vi "UDP Sender.vi"(4 "error in":errorcluster, 5 "Show panel":bool, 6 "boost":dbl=1.0, 7 "Spot Params":T1=[{"Intensity"=1.0, "Vortex"=0.0, "Phase"=0.0, "X"=4.0, "Y"=0.0, "Z"=0.0}, {"Intensity"=0.0, "Vortex"=0.0, "Phase"=0.0, "X"=-7.0, "Y"=6.0, "Z"=0.0}] {"Z" format="%_4g"; "Y" format="%_4g"; "X" format="%_4g"; "Phase" format="%_4g"; "Intensity" format="%_4g"}) -> (0 "error out":errorcluster, 3 "length":i32=234)   [LabVIEW 2020]
doc: "This VI sends UDP packets to the hologram server so that it can display holograms. It also has a lot of settings on the front panel, which control most of the aspects of hologram generation and display."
uses:
  <vilib>/Analysis/Matrix/Datatypes/RealMatrix.ctl
  _Controls/Spot Params.ctl
  <vilib>/Analysis/Matrix/NI_Matrix.lvlib
panel:
  in  "NA Position":cluster{"x":dbl, "y":dbl, "r":dbl}={"x"=0.0, "y"=0.0, "r"=1.0}
  in  "Save settings to defaults file":bool
  in  "SLM Settings":T2(tab)=enum."Scaling Factors"
  in  "Remote Host":string="127.0.0.1"
  in  "Local Port":u16=61556
  in  "Remote Port":u16=61557
  in  "-¹..¹ range control":enum16{"wrap round", "cast to range"}(ring)=enum."cast to range"
  out "'blazing function'":cluster{dbl, dbl}[](graph)=[{-3.141592653589793, 0.0}, {-2.938909256584, 0.057923902564858604}, {-2.736225859578207, 0.11496236941997928}, {-2.533542462572414, 0.1702299648556241}, {-2.330859065566621, 0.22284125316205516}, {-2.1281756685608277, 0.2719107986295345}, {-1.9254922715550344, 0.31655316554832424}, {-1.7228088745492414, 0.3558829182086864}, {-1.5201254775434483, 0.38901462090088307}, {-1.317442080537655, 0.41506283791517634}, {-1.114758683531862, 0.4334376236022463}, {-0.9120752865260688, 0.44502212608587055}, {-0.7093918895202758, 0.4511576344794046}, {-0.5067084925144827, 0.4531855832933398}, {-0.3040250955086896, 0.45244740703816744}, {-0.10134169850289654, 0.4502845402243789}, {0.10134169850289654, 0.44803841736246536}, {0.30402509550868917, 0.44705047296291806}, {0.5067084925144831, 0.44866214153622835}, {0.7093918895202758, 0.45421485759288766}, {0.9120752865260693, 0.46505005564338703}, {1.1147586835318615, 0.48250917019821804}, {1.3174420805376554, 0.5079336357678718}, {1.5201254775434485, 0.5426266162553631}, {1.7228088745492416, 0.5867222378526288}, {1.9254922715550338, 0.6389982972954518}, {2.1281756685608277, 0.6981566028735295}, {2.330859065566621, 0.7628989628765593}, {2.533542462572414, 0.8319271855942384}, {2.736225859578207, 0.9039430793162642}, {2.938909256584, 0.9776484523323339}, {3.141592653589793, 1.0}]
  in  "Hologram location on-screen":T3={"Display Mode"=0, "Coordinates (x,y,width,height)"=[2560, 0, 512, 512]} {"Display Mode" items=["Coordinates given below", "All of monitor 1", "All of monitor 2", "All of monitor 3", "All of monitor 4", "All of monitor 5"]}
  in  "Aspect Ratio and Centering":T4={"Physical Aspect Ratio (width/height)"=1.0, "Screen Aspect Ratio (width in pixels/height in pixels)"=1.0, "Illumination Centre (range: 0 to 1)"={"x"=0.49, "y"=0.52}} {"Illumination Centre (range: 0 to 1)"."y" min=0.0 max=1.0 step=0.001; "Illumination Centre (range: 0 to 1)"."x" min=0.0 max=1.0 step=0.001}
  in  "Zernike Coefficients":dbl[](array[numeric])=[1.0, 0.0, -1.0, 0.0, 0.0, 0.0, 0.0, 0.0, 0.0, 0.0, 0.0, 0.0]
  in  "Enable":bool=TRUE
  in  "Multiplier":dbl=10.0
  out "Phase Map":dbl[][](graph)=[[1.1504440784612413, 1.1088207694081724, 0.9839508422489622, 0.7758342969836143, 0.484471133612125, 0.10986135213450154, -0.3479950474492668, -0.8890980651391764, -1.5134477009352203, -2.2210439548374055, -3.0118868268457284, 2.39720899021939, 1.439872881998788, 0.39929015567204473, -0.7245391887608363, -1.9316151512998605, 3.0612475752345656, 1.6876783764832677, 0.23086255962582847, -1.3091998753377538, -2.932508928407473, 1.6441207075962554, -0.1456815816857464, -2.0187304890738824, 2.308159292611429, 0.2686171490110141, -1.8541716126955379, 2.222978314671346, -0.06630368324748659, -2.438832299272459, 1.38857777377601, -1.1504440784612413], [-1.38857777377601, -1.3469544647229412, -1.38857777377601, -1.5134477009352203, -1.7215642462005682, -2.0129274095720575, -2.387537191049681, -2.8453935906334493, 2.8966886988562273, 2.2723390630601834, 1.5647428091579982, 0.7738999371496718, -0.1001895529647907, -1.0575256611853927, -2.098108387512136, 3.0612475752345656, 1.8541716126955432, 0.5638490320503848, -0.8097201667009148, -2.2665359835583576, 2.476586888657649, 0.8532778355879307, -0.8532778355879307, -2.643080124869927, 1.767056274921524, -0.1892392505727507, -2.2287813941731667, 1.9316151512998587, -0.27442022851283454, -2.563702226431669, 1.3469544647229412, -1.1088207694081724], [2.438832299272459, 2.563702226431669, 2.6053255354847416, 2.563702226431669, 2.438832299272459, 2.230715754007111, 1.9393525906356253, 1.5647428091579947, 1.10688640957423, 0.5657833918843238, -0.05856624391172183, -0.766162497813907, -1.5570053698222317, -2.431094859936694, 2.8947543390222865, 1.8541716126955432, 0.7303422682626604, -0.4767336942763585, -1.7670562749215186, -3.1406254736728236, 1.6857440166493252, 0.1456815816857464, -1.477627471383978, 3.099002164619751, 1.3091998753377556, -0.5638490320503795, -2.520144557544656, 1.723498606034509, -0.39929015567204296, -2.605325535484738, 1.38857777377601, -0.9839508422489622], [0.06630368324748659, 0.27442022851283454, 0.39929015567204473, 0.44091346472511006, 0.3992901556720412, 0.27442022851283454, 0.06630368324748659, -0.22505948012400268, -0.5996692616016315, -1.0575256611853963, -1.5986286788753024, -2.222978314671348, -2.930574568573535, 2.5617678665977284, 1.6876783764832641, 0.7303422682626604, -0.31024045806408296, -1.434069802496964, -2.6411457650359838, 2.351716961498438, 0.9781477627471382, -0.478668054110301, -2.0187304890738833, 2.6411457650359846, 0.9345900938601268, -0.8552121954218688, -2.7282611028100057, 1.5986286788753006, -0.44091346472511184, -2.5637022264316656, 1.5134477009352203, -0.7758342969836143], [-2.222978314671346, -1.9316151512998587, -1.723498606034509, -1.5986286788753006, -1.5570053698222317, -1.5986286788753006, -1.7234986060345108, -1.9316151512998587, -2.222978314671346, -2.597588096148975, -3.05544449573274, 2.6866377937569386, 2.062288157960893, 1.3546919040587078, 0.5638490320503848, -0.31024045806408296, -1.267576566284685, -2.3081592926114256, 2.8511966701352787, 1.6441207075962545, 0.35379812695109436, -1.0197710718002062, -2.476586888657649, 2.2665359835583576, 0.6432269304886411, -1.063328740687215, -2.8531310299692105, 1.5570053698222317, -0.3992901556720412, -2.438832299272459, 1.7215642462005682, -0.484471133612125], [1.8541716126955468, 2.228781394173174, 2.5201445575446613, 2.728261102810009, 2.8531310299692194, 2.8947543390222883, 2.8531310299692194, 2.728261102810009, 2.5201445575446613, 2.228781394173174, 1.854171612695545, 1.3963152131117766, 0.8552121954218705, 0.2308625596258267, -0.4767336942763585, -1.267576566284685, -2.1416660563991483, -3.099002164619751, 2.1436004162330935, 1.019771071800208, -0.18730489073881262, -1.4776274713839723, -2.8511966701352773, 1.9751728201868701, 0.4351103852232914, -1.188198667846426, -2.894754339022281, 1.5986286788753006, -0.27442022851283454, -2.230715754007111, 2.0129274095720575, -0.10986135213450154], [-0.2686171490110123, 0.18923925057275603, 0.5638490320503831, 0.8552121954218705, 1.0633287406872185, 1.1881986678464287, 1.2298219768994976, 1.1881986678464287, 1.0633287406872185, 0.8552121954218705, 0.5638490320503813, 0.18923925057275426, -0.2686171490110123, -0.8097201667009166, -1.434069802496964, -2.141666056399149, -2.932508928407474, 2.47658688865765, 1.519250780437047, 0.47866805411030144, -0.6451612903225801, -1.8522372528616007, 3.14062547367282, 1.7670562749215213, 0.31024045806408207, -1.2298219768994958, -2.8531310299692123, 1.7234986060345108, -0.06630368324748659, -1.9393525906356235, 2.387537191049681, 0.3479950474492668], [-2.308159292611429, -1.767056274921524, -1.3091998753377556, -0.9345900938601268, -0.6432269304886411, -0.4351103852232914, -0.31024045806408296, -0.2686171490110123, -0.31024045806408296, -0.4351103852232914, -0.6432269304886411, -0.9345900938601286, -1.3091998753377556, -1.7670562749215213, -2.3081592926114283, -2.932508928407474, 2.643080124869927, 1.8522372528616033, 0.97814776274714, 0.020811654526533996, -1.0197710718002075, -2.143600416233089, 2.932508928407472, 1.642186347762312, 0.2686171490110123, -1.188198667846426, -2.728261102810004, 1.9316151512998587, 0.22505948012400268, -1.564742809157993, 2.8453935906334493, 0.8890980651391764], [2.0187304890738824, 2.643080124869927, -3.099002164619751, -2.6411457650359846, -2.2665359835583576, -1.9751728201868701, -1.7670562749215213, -1.642186347762312, -1.6005630387092422, -1.642186347762312, -1.7670562749215222, -1.9751728201868701, -2.2665359835583576, -2.6411457650359855, -3.099002164619752, 2.643080124869927, 2.0187304890738815, 1.3111342351716972, 0.5202913631633734, -0.3537981269510926, -1.311134235171696, -2.3517169614984375, 2.8076390012482637, 1.6005630387092422, 0.31024045806408296, -1.0633287406872167, -2.520144557544656, 2.222978314671346, 0.5996692616016315, -1.1068864095742263, -2.896688698856229, 1.5134477009352203], [0.1456815816857464, 0.8532778355879307, 1.477627471383978, 2.0187304890738833, 2.476586888657649, 2.851196670135277, -3.14062547367282, -2.932508928407472, -2.8076390012482637, -2.766015692195194, -2.8076390012482637, -2.932508928407473, -3.140625473672822, 2.851196670135277, 2.476586888657649, 2.0187304890738815, 1.4776274713839754, 0.8532778355879307, 0.14568158168574596, -0.645161290322581, -1.5192507804370443, -2.4765868886576468, 2.766015692195194, 1.642186347762312, 0.4351103852232914, -0.8552121954218688, -2.2287813941731685, 2.597588096148975, 1.0575256611853963, -0.565783391884322, -2.2723390630601834, 2.2210439548374055], [-1.6441207075962527, -0.8532778355879289, -0.14568158168574463, 0.4786680541103028, 1.019771071800208, 1.4776274713839754, 1.8522372528616033, 2.143600416233091, 2.3517169614984397, 2.476586888657648, 2.5182101977107187, 2.476586888657648, 2.3517169614984397, 2.1436004162330917, 1.8522372528616025, 1.4776274713839754, 1.0197710718002089, 0.4786680541103028, -0.14568158168574197, -0.8532778355879294, -1.6441207075962532, -2.5182101977107165, 2.8076390012482637, 1.7670562749215222, 0.6432269304886402, -0.5638490320503804, -1.8541716126955414, 3.05544449573274, 1.5986286788753024, 0.05856624391172538, -1.5647428091579982, 3.01188682684573], [2.932508928407473, -2.476586888657649, -1.6857440166493252, -0.9781477627471382, -0.35379812695109436, 0.18730489073881262, 0.6451612903225801, 1.019771071800207, 1.3111342351716964, 1.5192507804370443, 1.6441207075962527, 1.6857440166493234, 1.6441207075962536, 1.5192507804370443, 1.3111342351716964, 1.019771071800208, 0.6451612903225805, 0.1873048907388144, -0.35379812695109125, -0.9781477627471387, -1.6857440166493232, -2.476586888657647, 2.932508928407473, 1.9751728201868701, 0.9345900938601286, -0.18923925057275248, -1.396315213111774, -2.6866377937569386, 2.222978314671348, 0.7661624978139105, -0.7738999371496718, -2.39720899021939], [1.3091998753377547, 2.2665359835583576, 3.1406254736728236, -2.3517169614984375, -1.644120707596254, -1.019771071800208, -0.47866805411030144, -0.020811654526533996, 0.3537981269510926, 0.645161290322581, 0.8532778355879294, 0.9781477627471382, 1.019771071800208, 0.9781477627471382, 0.8532778355879294, 0.645161290322581, 0.35379812695109303, -0.02081165452653444, -0.478668054110301, -1.019771071800208, -1.6441207075962536, -2.351716961498438, 3.140625473672822, 2.2665359835583576, 1.3091998753377556, 0.2686171490110141, -0.8552121954218679, -2.062288157960893, 2.930574568573535, 1.5570053698222335, 0.1001895529647907, -1.439872881998788], [-0.23086255962582225, 0.8097201667009184, 1.767056274921524, 2.641145765035988, -2.8511966701352747, -2.14360041623309, -1.5192507804370434, -0.9781477627471373, -0.5202913631633708, -0.14568158168574374, 0.14568158168574463, 0.3537981269510935, 0.47866805411030233, 0.5202913631633721, 0.47866805411030233, 0.35379812695109303, 0.1456815816857442, -0.1456815816857433, -0.5202913631633703, -0.9781477627471387, -1.5192507804370448, -2.14360041623309, -2.851196670135277, 2.6411457650359855, 1.7670562749215213, 0.8097201667009193, -0.23086255962582314, -1.3546919040587078, -2.5617678665977284, 2.431094859936696, 1.0575256611853927, -0.39929015567204473], [-1.687678376483266, -0.5638490320503831, 0.47673369427636114, 1.4340698024969658, 2.3081592926114274, 3.099002164619753, -2.4765868886576476, -1.8522372528616018, -1.3111342351716964, -0.8532778355879298, -0.4786680541103019, -0.1873048907388135, 0.020811654526534884, 0.1456815816857442, 0.18730489073881396, 0.1456815816857442, 0.020811654526534884, -0.1873048907388135, -0.478668054110301, -0.8532778355879294, -1.311134235171696, -1.852237252861602, -2.476586888657649, 3.099002164619752, 2.3081592926114283, 1.4340698024969658, 0.47673369427636203, -0.563849032050384, -1.6876783764832641, -2.8947543390222865, 2.098108387512136, 0.7245391887608363], [-3.0612475752345656, -1.8541716126955432, -0.7303422682626612, 0.31024045806408207, 1.267576566284684, 2.1416660563991483, 2.932508928407474, -2.6430801248699276, -2.018730489073882, -1.4776274713839759, -1.0197710718002084, -0.6451612903225805, -0.35379812695109303, -0.1456815816857442, -0.020811654526534884, 0.020811654526534884, -0.020811654526534884, -0.14568158168574374, -0.35379812695109214, -0.645161290322581, -1.019771071800208, -1.4776274713839743, -2.018730489073882, -2.6430801248699276, 2.932508928407474, 2.141666056399151, 1.2675765662846876, 0.31024045806408207, -0.7303422682626595, -1.8541716126955414, -3.0612475752345656, 1.9316151512998605], [1.9316151512998605, -3.0612475752345656, -1.8541716126955432, -0.7303422682626595, 0.31024045806408207, 1.267576566284684, 2.141666056399149, 2.932508928407474, -2.6430801248699276, -2.018730489073882, -1.477627471383975, -1.019771071800208, -0.645161290322581, -0.35379812695109303, -0.1456815816857442, -0.020811654526534884, 0.020811654526534884, -0.020811654526534884, -0.14568158168574374, -0.35379812695109303, -0.6451612903225805, -1.019771071800208, -1.4776274713839759, -2.018730489073882, -2.6430801248699276, 2.932508928407474, 2.14166605639915, 1.267576566284684, 0.31024045806408207, -0.7303422682626604, -1.8541716126955432, -3.0612475752345656], [0.7245391887608381, 2.098108387512138, -2.8947543390222847, -1.6876783764832624, -0.5638490320503822, 0.47673369427636025, 1.434069802496965, 2.308159292611429, 3.099002164619753, -2.476586888657648, -1.8522372528616025, -1.3111342351716955, -0.8532778355879289, -0.4786680541103019, -0.18730489073881396, 0.020811654526534884, 0.14568158168574374, 0.1873048907388135, 0.14568158168574374, 0.02081165452653444, -0.1873048907388144, -0.47866805411030233, -0.8532778355879307, -1.3111342351716975, -1.8522372528616033, -2.4765868886576485, 3.099002164619753, 2.3081592926114256, 1.434069802496964, 0.47673369427636025, -0.5638490320503848, -1.6876783764832677], [-0.39929015567204296, 1.0575256611853963, 2.4310948599366977, -2.5617678665977266, -1.354691904058706, -0.23086255962582491, 0.8097201667009202, 1.767056274921524, 2.6411457650359864, -2.851196670135276, -2.14360041623309, -1.5192507804370439, -0.9781477627471382, -0.5202913631633721, -0.1456815816857442, 0.14568158168574374, 0.35379812695109214, 0.478668054110301, 0.5202913631633708, 0.478668054110301, 0.35379812695109125, 0.14568158168574286, -0.14568158168574596, -0.5202913631633734, -0.9781477627471404, -1.5192507804370456, -2.143600416233091, -2.8511966701352787, 2.6411457650359838, 1.7670562749215186, 0.8097201667009148, -0.23086255962582847], [-1.439872881998788, 0.1001895529647907, 1.5570053698222317, 2.930574568573535, -2.062288157960893, -0.8552121954218714, 0.2686171490110123, 1.3091998753377556, 2.2665359835583576, 3.140625473672822, -2.3517169614984397, -1.6441207075962536, -1.019771071800208, -0.47866805411030233, -0.020811654526534884, 0.35379812695109303, 0.645161290322581, 0.8532778355879289, 0.9781477627471382, 1.019771071800208, 0.9781477627471382, 0.8532778355879298, 0.645161290322581, 0.3537981269510926, -0.020811654526533996, -0.47866805411030056, -1.0197710718002062, -1.644120707596254, -2.3517169614984375, 3.1406254736728236, 2.2665359835583576, 1.3091998753377547], [-2.39720899021939, -0.7738999371496718, 0.766162497813907, 2.222978314671348, -2.6866377937569386, -1.3963152131117775, -0.18923925057275426, 0.9345900938601286, 1.9751728201868701, 2.932508928407473, -2.4765868886576485, -1.6857440166493232, -0.9781477627471387, -0.3537981269510935, 0.1873048907388135, 0.6451612903225805, 1.019771071800208, 1.3111342351716955, 1.5192507804370443, 1.6441207075962536, 1.6857440166493234, 1.6441207075962536, 1.5192507804370443, 1.3111342351716964, 1.019771071800207, 0.6451612903225805, 0.1873048907388144, -0.35379812695109436, -0.9781477627471382, -1.6857440166493234, -2.476586888657649, 2.932508928407473], [3.011886826845732, -1.5647428091579982, 0.0585662439117236, 1.5986286788753041, 3.0554444957327433, -1.854171612695545, -0.5638490320503813, 0.6432269304886402, 1.7670562749215222, 2.8076390012482637, -2.5182101977107183, -1.6441207075962536, -0.8532778355879298, -0.14568158168574508, 0.478668054110301, 1.019771071800208, 1.4776274713839745, 1.8522372528616007, 2.143600416233089, 2.351716961498438, 2.476586888657647, 2.518210197710717, 2.4765868886576463, 2.351716961498438, 2.143600416233089, 1.8522372528616016, 1.4776274713839737, 1.0197710718002062, 0.478668054110301, -0.14568158168574463, -0.8532778355879307, -1.6441207075962554], [2.2210439548374055, -2.2723390630601834, -0.5657833918843238, 1.0575256611853963, 2.597588096148975, -2.228781394173174, -0.8552121954218705, 0.4351103852232914, 1.642186347762312, 2.766015692195194, -2.4765868886576485, -1.5192507804370443, -0.645161290322581, 0.14568158168574374, 0.8532778355879298, 1.4776274713839754, 2.0187304890738815, 2.476586888657648, 2.851196670135276, -3.140625473672822, -2.932508928407473, -2.8076390012482637, -2.766015692195194, -2.8076390012482637, -2.932508928407472, -3.14062547367282, 2.851196670135277, 2.476586888657649, 2.0187304890738833, 1.4776274713839772, 0.8532778355879307, 0.1456815816857464], [1.5134477009352203, -2.896688698856229, -1.10688640957423, 0.5996692616016315, 2.222978314671346, -2.5201445575446613, -1.0633287406872194, 0.31024045806408296, 1.6005630387092422, 2.8076390012482637, -2.3517169614984392, -1.311134235171696, -0.3537981269510926, 0.5202913631633708, 1.3111342351716964, 2.0187304890738815, 2.643080124869927, -3.099002164619753, -2.6411457650359864, -2.2665359835583576, -1.9751728201868701, -1.7670562749215222, -1.642186347762312, -1.6005630387092422, -1.642186347762312, -1.7670562749215204, -1.9751728201868683, -2.2665359835583576, -2.6411457650359846, -3.099002164619752, 2.643080124869927, 2.0187304890738824], [0.8890980651391764, 2.8453935906334493, -1.5647428091579965, 0.22505948012400268, 1.9316151512998587, -2.728261102810009, -1.1881986678464278, 0.2686171490110123, 1.642186347762312, 2.932508928407472, -2.143600416233091, -1.0197710718002075, 0.020811654526533996, 0.9781477627471373, 1.8522372528616016, 2.643080124869927, -2.932508928407474, -2.308159292611429, -1.767056274921524, -1.3091998753377556, -0.9345900938601286, -0.6432269304886411, -0.4351103852232914, -0.31024045806408296, -0.2686171490110123, -0.31024045806408296, -0.4351103852232914, -0.6432269304886411, -0.9345900938601268, -1.3091998753377556, -1.767056274921524, -2.308159292611429], [0.34799504744927034, 2.3875371910496845, -1.9393525906356235, -0.06630368324748481, 1.7234986060345108, -2.8531310299692194, -1.2298219768994976, 0.31024045806408207, 1.7670562749215204, 3.14062547367282, -1.8522372528616033, -0.6451612903225805, 0.47866805411030056, 1.5192507804370425, 2.4765868886576463, -2.932508928407474, -2.141666056399151, -1.4340698024969658, -0.809720166700922, -0.2686171490110141, 0.18923925057275248, 0.5638490320503813, 0.8552121954218688, 1.0633287406872167, 1.1881986678464251, 1.2298219768994958, 1.1881986678464251, 1.063328740687215, 0.8552121954218688, 0.5638490320503813, 0.1892392505727507, -0.2686171490110141], [-0.10986135213449799, 2.0129274095720575, -2.2307157540071127, -0.27442022851283454, 1.5986286788753024, -2.8947543390222883, -1.1881986678464278, 0.4351103852232914, 1.9751728201868683, -2.8511966701352773, -1.4776274713839763, -0.1873048907388144, 1.0197710718002062, 2.143600416233088, -3.0990021646197548, -2.14166605639915, -1.2675765662846885, -0.4767336942763638, 0.23086255962581959, 0.855212195421867, 1.396315213111773, 1.8541716126955397, 2.2287813941731685, 2.520144557544656, 2.728261102810004, 2.8531310299692123, 2.894754339022283, 2.8531310299692105, 2.7282611028100057, 2.520144557544654, 2.2287813941731667, 1.8541716126955379], [-0.484471133612125, 1.7215642462005682, -2.4388322992724607, -0.3992901556720412, 1.5570053698222317, -2.8531310299692194, -1.0633287406872185, 0.6432269304886411, 2.2665359835583576, -2.476586888657649, -1.019771071800208, 0.35379812695109436, 1.6441207075962545, 2.851196670135275, -2.3081592926114274, -1.267576566284685, -0.31024045806408296, 0.5638490320503813, 1.354691904058706, 2.062288157960893, 2.6866377937569386, -3.0554444957327433, -2.597588096148975, -2.222978314671346, -1.9316151512998587, -1.7234986060345108, -1.5986286788753024, -1.5570053698222317, -1.5986286788753006, -1.7234986060345108, -1.9316151512998587, -2.222978314671346], [-0.7758342969836143, 1.5134477009352203, -2.563702226431671, -0.44091346472511184, 1.5986286788753006, -2.728261102810009, -0.8552121954218714, 0.9345900938601268, 2.6411457650359846, -2.0187304890738833, -0.4786680541103028, 0.9781477627471382, 2.351716961498438, -2.641145765035988, -1.4340698024969658, -0.31024045806408296, 0.7303422682626604, 1.6876783764832624, 2.5617678665977266, -2.930574568573535, -2.222978314671348, -1.5986286788753041, -1.0575256611853963, -0.5996692616016315, -0.22505948012400268, 0.06630368324748481, 0.27442022851283454, 0.3992901556720412, 0.44091346472511006, 0.3992901556720412, 0.27442022851283454, 0.06630368324748659], [-0.9839508422489622, 1.38857777377601, -2.6053255354847416, -0.3992901556720412, 1.7234986060345108, -2.5201445575446613, -0.5638490320503831, 1.3091998753377556, 3.099002164619752, -1.4776274713839772, 0.14568158168574286, 1.6857440166493234, -3.1406254736728236, -1.7670562749215248, -0.47673369427636203, 0.7303422682626604, 1.8541716126955414, 2.8947543390222847, -2.4310948599366995, -1.5570053698222335, -0.7661624978139105, -0.05856624391172538, 0.5657833918843203, 1.1068864095742263, 1.5647428091579947, 1.9393525906356217, 2.2307157540071074, 2.438832299272459, 2.5637022264316656, 2.605325535484738, 2.563702226431669, 2.438832299272459], [-1.1088207694081724, 1.3469544647229412, -2.563702226431669, -0.27442022851283454, 1.9316151512998587, -2.228781394173174, -0.18923925057275603, 1.767056274921524, -2.643080124869927, -0.8532778355879307, 0.8532778355879289, 2.476586888657649, -2.2665359835583576, -0.8097201667009184, 0.5638490320503831, 1.8541716126955432, 3.0612475752345656, -2.098108387512138, -1.0575256611853963, -0.1001895529647907, 0.7738999371496718, 1.5647428091579982, 2.2723390630601834, 2.8966886988562273, -2.8453935906334493, -2.3875371910496845, -2.0129274095720575, -1.7215642462005682, -1.5134477009352203, -1.38857777377601, -1.3469544647229412, -1.38857777377601], [-1.1504440784612413, 1.38857777377601, -2.438832299272459, -0.06630368324748659, 2.222978314671346, -1.8541716126955468, 0.2686171490110123, 2.308159292611429, -2.0187304890738824, -0.1456815816857464, 1.6441207075962527, -2.932508928407473, -1.3091998753377538, 0.23086255962582314, 1.687678376483266, 3.0612475752345656, -1.9316151512998605, -0.7245391887608381, 0.39929015567204473, 1.439872881998788, 2.39720899021939, -3.011886826845732, -2.2210439548374055, -1.5134477009352203, -0.8890980651391764, -0.34799504744927034, 0.10986135213449799, 0.484471133612125, 0.7758342969836143, 0.9839508422489622, 1.1088207694081724, 1.1504440784612413]]
  in  "SLM Transformation Matrix":T5=[[-1.8400000000000003e-05, 0.0, 0.0], [0.0, 1.8599999999999998e-05, 0.0], [0.0, 0.0, -1.6310000000000005e-05]]
  out "message":string="<data>\n<spots>\n  0.000000E+0 7.440000E-5 0.000000E+0 1.000000 0 0.000000 0.000000 0.000000 1.000000\r\n  -1.104000E-4 -1.302000E-4 0.000000E+0 0.000000 0 0.000000 0.000000 0.000000 1.000000\r\n\n</spots>\n<totalA>\n1.000000\n</totalA>\n</data>"
  # "Network Settings:\nIn order for this program to display a hologram on the SLM, the SLM server must be running.  Use either the \"hologram_server.exe\" program, or the LabView alternative.  Note that the hologram_server.exe program will only run on relatively recent graphics cards; the LabView version is unsupported, we reccommend all users purchase a recent graphics card (even a relatively inexpensive one) to take advantage of the order-of-magnitude increase in performance.  The port settings should be left as-is (local 61556, remote 61557) and the remote host should be 127.0.0.1 if the server is running on this machine.\n\nIf you are running the server on a different machine, enter the other machine's IP address in the \"remote host\" field.  It's best to have them on the same subnet, preferably connected to the same hub/switch."
  # "Blazing Function\nThis curve controls the output level (0=black, 1=white) for a given phase on the SLM.  It can be used to optimise the hologram to direct as much light as possible into the first diffraction order, and is particularly useful when the SLM has a range of more or less than one wavelength."
  # "Position of SLM Output Window\nThis determines where the hologram image is shown; usually \"all monitor 2\" is the right one, displaying the hologram full-screen on the second monitor.  You can enter coordinates manually if you need finer control.  By default, the hologram generated is square and the output window will be \"letterboxed\", showing solid black on the outside, and having the hologram in the central square (which will fill either the width or the height of the window, whichever is smaller).\n\nFor Hamamatsu SLMs, this is the correct behaviour for all the models we've tested.\nFor Holoeye SLMs, this is also correct, but it does mean you need to be using the centre of the SLM, not the sides.\nFor Boulder SLMs, you may need to use the coordinates to place the window in the top left corner of the SLM screen."
  # "Aspect ratios and Centering\nThe Physical aspect ratio should be the width of the hologram in the real world divided by its height, while the screen aspect ratio refers to its dimensions in pixels.  Most SLMs have square pixels, so these values should both be the same if the whole SLM is to be used.  NB that using a value of 1 is usually correct even if the SLM is non-square, as a square hologram will give more symmetric spots.  It is OK to use a square aspect ratio even if the hologram's size in pixels is not square; the edges of the area will simply be filled in black.\n\nIf the illumination of the SLM is off-centre, moving a spot in Z will also affect its position in X and Y (think of an off-centre lens).  The \"illumination centre\" can correct for this.  Setting this parameter correctly is particularly important if Laguerre-Gauss beams are to be used (i.e. spots with L not equal to 0).  The real centre of the hologram is at 0.5,0.5."
  # "Aberration Correction\nThe engine allows Zernike polynomials to be added to the hologram to compensate for aberrations.  The coefficients can be adjusted here.  The polynomials included are the first 15, ignoring piston and tilt (as these are adjusted for each spot)."
  # "Astig"
  # "Defocus"
  # "Astig"
  # "Tirefoil"
  # "Coma"
  # "Coma"
  # "Tirefoil"
  # "Tirefoil"
  # "Astig"
  # "Spher"
  # "Astig"
  # "Tirefoil"
  # "Scaling Factors\nTo translate between the coordinates used in the rest of the program and the numbers we send to the SLM, it's necessary to scale things.  The control below is a matrix, to allow maximum flexibility when setting up a system- it's useful if, for example, either your SLM or camera is mounted on its side (so x and y are swapped).\n\nMost people can ignore the matrix and just use the 3 diagonal elements for scaling values for X,Y and Z.  Between about 10 and 100 tends to be best (and negative values are sometimes correct)."
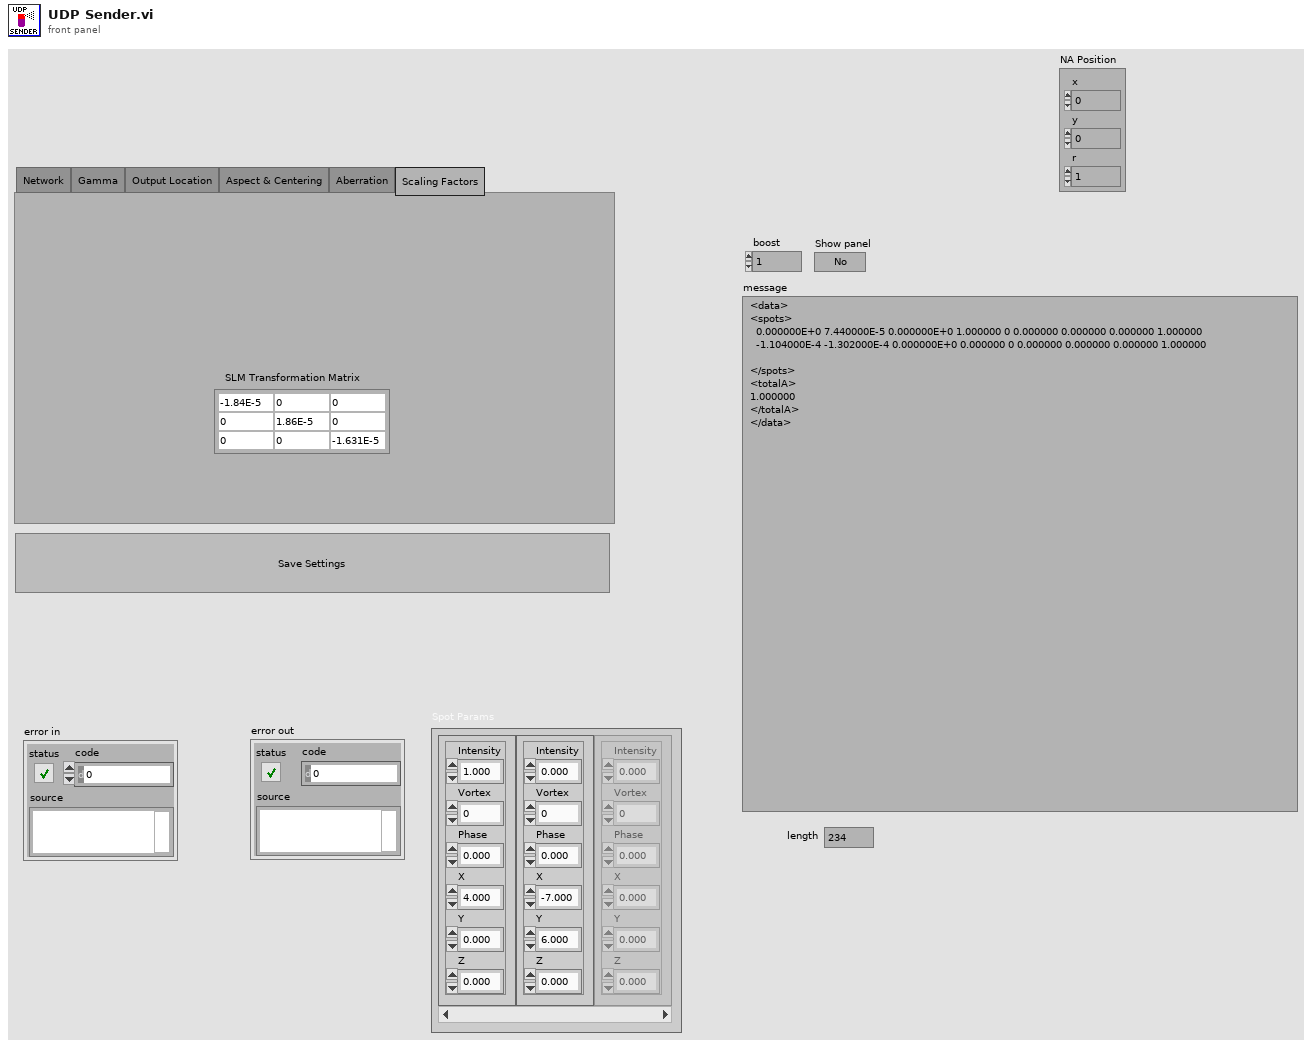
[diagram p1: front panel]
types:
  T1 = typedef "Spot Params.ctl" = cluster{"Intensity":dbl, "Vortex":dbl, "Phase":dbl, "X":dbl, "Y":dbl, "Z":dbl}[]
  T2 = enum32{"Network", "Gamma", "Output Location", "Aspect & Centering", "Aberration", "Scaling Factors"}
  T3 = cluster{"Display Mode":u16, "Coordinates (x,y,width,height)":i32[]}
  T4 = cluster{"Physical Aspect Ratio (width/height)":dbl, "Screen Aspect Ratio (width in pixels/height in pixels)":dbl, "Illumination Centre (range: 0 to 1)":cluster{"x":dbl, "y":dbl}}
  T5 = typedef "NI_Matrix.lvlib/RealMatrix.ctl" = dbl[][]
  T6 = typedef "LVCursorListTypeDef.ctl" = cluster{"Name":string, "Color":u32, "Style":u8, "Point Style":u8, "Name Visible":bool, "Allow Drag":bool, "Cursor Mode":u32, "Plot":i32, "Index":i32, "Position":cluster{"X":dbl, "Y":dbl}, "X Scale":u32, "Y Scale":u32, "Watch Plots":i32[], "Watch All Plots":bool, "Plot Area":i32, "Label Offset":cluster{"X":dbl, "Y":dbl}}[]
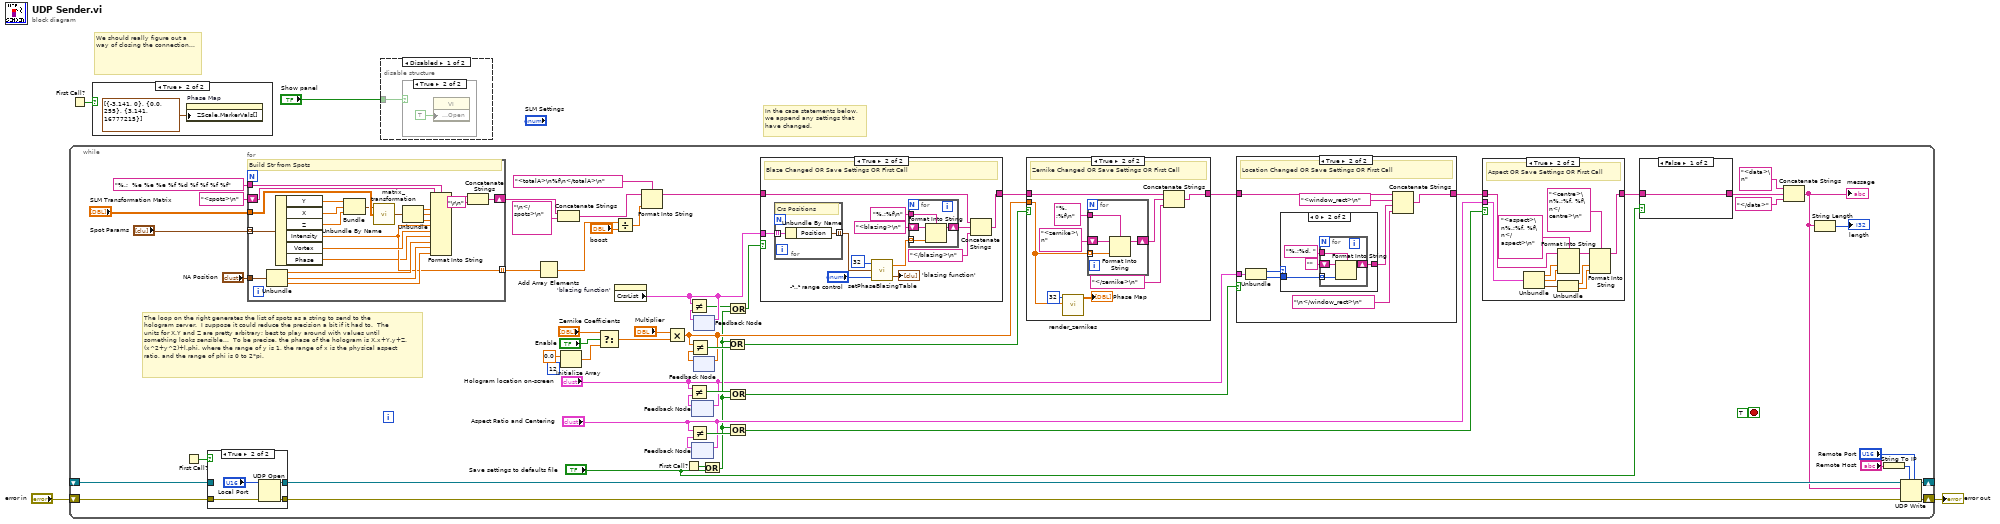
[diagram p0: block diagram]
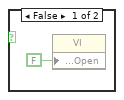
[diagram p2: hidden frame]
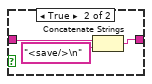
[diagram p6: hidden frame]
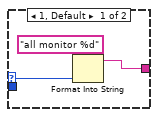
[diagram p8: hidden frame]
diagram:
  # "In the case statements below, we append any settings that have changed."
  # "We should really figure out a way of closing the connection..."
  n1 = First Call?() -> (First Call?: T/F=w3:bool)
  n2 = while {
    shift-right: [w61] -> _
    shift-left: _ -> [w60]
    shift-right: [w62] -> w2
    shift-left: "error in" -> [w59]
    stop <- TRUE stop-if-true
    # "The loop on the right generates the list of spots as a string to send to the hologram server.  I suppose it could reduce the precision a bit if it had to.  The units for X,Y and Z are pretty arbitrary; best to play around with values until something looks sensible...  To be precise, the phase of the hologram is X.x+Y.y+Z.(x^2+y^2)+l.phi, where the range of y is 1, the range of x is the physical aspect ratio, and the range of phi is 0 to 2*pi."
    n3 = First Call?() -> (First Call?: T/F=w40:bool)
    n4 = case shown="True" w40 {
      tunnel: [w157 w160] -> w58
      tunnel: [w156 w159] -> w56
      tunnel: w60 -> [w157 _]
      tunnel: w59 -> [w156 w158]
      frame False {
      }
      frame True {
        n5 = UDP Open(8:w158, 11:"Local Port") -> (port=w160:refnum<k16>, 0:w159:errorcluster)  [unwired: 4 out]
      }
    }
    n6 = for {
      tunnel: "Spot Params" -> [w140] mode=indexing
      shift-right: [w152] -> w55
      shift-left: "<spots>\n" ("Data String") -> [w155]
      tunnel: "%.;  %e %e %e %f %d %f %f %f %f" ("initial string") -> [w154]
      tunnel: "SLM Transformation Matrix" -> [w150]
      tunnel: [w144] -> w32 mode=indexing
      tunnel: "NA Position" -> [w139]
      # "Build Str from Spots"
      n7 = Unbundle(w139) -> ("x"=w148:dbl, "y"=w147:dbl, "r"=w146:dbl)
      n8 = Unbundle By Name(w140) -> ("Y"=w137:dbl, "X"=w136:dbl, "Z"=w135:dbl, "Intensity"=w144:dbl, "Vortex"=w149:dbl, "Phase"=w138:dbl)
      n9 = Bundle("Y"=w137, "X"=w136, "Z"=w135) -> (w134:cluster{"Y":dbl, "X":dbl, "Z":dbl})  [unwired: 1 in]
      n10 = call "matrix_transformation.vi"("Transformation Matrix"=w150, "Input Vector"=w134) -> ("Output Vector"=w143:cluster{dbl, dbl, dbl})  [unwired: 2 in]
      n11 = Unbundle(w143) -> (w142:dbl, w141:dbl, w151:dbl)
      n12 = Format Into String(format string=w154, initial string=w155, w142, w141, w151, w144, w149, w138, w148, w147, w146) -> (resulting string=w145:string)  [unwired: 1 in, 1 out]
      n13 = Concatenate Strings(w145, "\r\n") -> (w152:string)
    }
    n14 = Add Array Elements(numeric array=w32) -> (sum=w31:dbl)
    n15 = Concatenate Strings(w55, "\n</spots>\n" ("Data String")) -> (w35:string)
    n16 = Initialize Array(0.0 ("element"), 12 ("dimension size")) -> (w25:dbl[])
    n17 = Select(t="Zernike Coefficients", s="Enable", f=w25) -> (s? t:f=w23:dbl[])
    n18 = Divide(x=w31, y="boost") -> (x/y=w34:dbl)
    n19 = property on="'blazing function'" class="XYGraph (strict)"() -> ("CrsrList"=w18:T6)  [unwired: 2 in, 2 out]
    n20 = Format Into String(format string="<totalA>\n%f\n</totalA>\n", initial string=w35, w34) -> (resulting string=w36:string)  [unwired: 1 in, 1 out]
    n21 = Multiply(x="Multiplier", y=w23) -> (x*y=w15:dbl[])
    n22 = First Call?() -> (First Call?: T/F=w16:bool)
    n23 = feedback-in #1("Hologram location on-screen") -> ()
    n24 = feedback #1() -> (w49:T3)  [unwired: 1 out]
    n25 = Not Equal?(x="Hologram location on-screen", y=w49) -> (x != y?=w13:bool)
    n26 = feedback-in #2("Aspect Ratio and Centering") -> ()
    n27 = feedback #2() -> (w44:T4)  [unwired: 1 out]
    n28 = Not Equal?(x="Aspect Ratio and Centering", y=w44) -> (x != y?=w43:bool)
    n29 = feedback-in #3(w18) -> ()
    n30 = feedback #3() -> (w39:T6)  [unwired: 1 out]
    n31 = Not Equal?(x=w18, y=w39) -> (x != y?=w17:bool)
    n32 = feedback-in #4(w15) -> ()
    n33 = feedback #4() -> (w14:dbl[])  [unwired: 1 out]
    n34 = Not Equal?(x=w15, y=w14) -> (x != y?=w28:bool)
    n35 = Or(x=w16, y="Save settings to defaults file") -> (x .or. y?=w12:bool)
    n36 = Or(x=w12, y=w28) -> (x .or. y?=w9:bool)
    n37 = Or(x=w17, y=w12) -> (x .or. y?=w51:bool)
    n38 = Or(x=w13, y=w12) -> (x .or. y?=w47:bool)
    n39 = Or(x=w12, y=w43) -> (x .or. y?=w11:bool)
    n40 = case shown="True" w51 {
      tunnel: w36 -> [w115 w116]
      tunnel: [w115 w124] -> w30
      tunnel: w18 -> [_ w118]
      frame False {
      }
      frame True {
        # "Blaze Changed OR Save Settings OR First Call"
        n41 = for {
          tunnel: w118 -> [w129] mode=indexing
          tunnel: [w128] -> w120 mode=indexing
          # "Crs Positions"
          n42 = Unbundle By Name(w129) -> ("Position"=w128:cluster{"X":dbl, "Y":dbl})
        }
        n43 = call "setPhaseBlazingTable.vi"("-¹..¹ range control"="-¹..¹ range control", "Anchor Points"=w120, "#elements (default 256)"=32) -> ("blazing graph"=→"'blazing function'":cluster{dbl, dbl}[], "blazing table"=w119:dbl[])
        n44 = for {
          shift-right: [w130] -> w125
          shift-left: "<blazing>\n" ("Data String") -> [w133]
          tunnel: "%.;%f\n" ("initial string") -> [w132]
          tunnel: w119 -> [w131] mode=indexing
          n45 = Format Into String(format string=w132, initial string=w133, w131) -> (resulting string=w130:string)  [unwired: 1 in, 1 out]
        }
        n46 = Concatenate Strings(w116, w125, "</blazing>\n" ("Data String")) -> (w124:string)
      }
    }
    n47 = case shown="True" w9 {
      tunnel: w30 -> [w65 w73]
      tunnel: [w65 w72] -> w29
      tunnel: w15 -> [_ w68]
      frame False {
      }
      frame True {
        # "Zernike Changed OR Save Settings OR First Call"
        n48 = call "render_zernikes.vi"("Size"=32, "Coefficients"=w68) -> ("Phase Map"=→"Phase Map":dbl[][])  [unwired: 6 in]
        n49 = for {
          shift-right: [w75] -> w70
          shift-left: "<zernike>\n" -> [w78]
          tunnel: "%.;%f\n" ("initial string") -> [w77]
          tunnel: w68 -> [w76] mode=indexing
          n50 = Format Into String(format string=w77, initial string=w78, w76) -> (resulting string=w75:string)  [unwired: 1 in, 1 out]
        }
        n51 = Concatenate Strings(w73, w70, "</zernike>\n" ("string")) -> (w72:string)
      }
    }
    n52 = case shown="True" w47 {
      tunnel: "Hologram location on-screen" -> [_ w91]
      tunnel: w29 -> [w83 w87]
      tunnel: [w83 w84] -> w46
      frame False {
      }
      frame True {
        # "Location Changed OR Save Settings OR First Call"
        n53 = Unbundle(w91) -> ("Display Mode"=w89:u16, "Coordinates (x,y,width,height)"=w90:i32[])
        n54 = case shown="0" w89 {
          selector: w89 -> [w94 _]
          tunnel: w90 -> [_ w95]
          tunnel: [w92 w96] -> w88
          frame 1, Default {
            n55 = Format Into String(format string="all monitor %d", w94) -> (resulting string=w92:string)  [unwired: 2 in, 1 out]
          }
          frame 0 {
            n56 = for {
              shift-right: [w99] -> w96
              shift-left: "" -> [w102]
              tunnel: "%.;%d, " ("initial string") -> [w101]
              tunnel: w95 -> [w100] mode=indexing
              n57 = Format Into String(format string=w101, initial string=w102, w100) -> (resulting string=w99:string)  [unwired: 1 in, 1 out]
            }
          }
        }
        n58 = Concatenate Strings(w87, "<window_rect>\n" ("Data String"), w88, "\n</window_rect>\n" ("Data String")) -> (w84:string)
      }
    }
    n59 = case shown="True" w11 {
      tunnel: w46 -> [w103 w109]
      tunnel: "Aspect Ratio and Centering" -> [_ w108]
      tunnel: [w103 w104] -> w38
      frame False {
      }
      frame True {
        # "Aspect OR Save Settings OR First Call"
        n60 = Unbundle(w108) -> ("Physical Aspect Ratio (width/height)"=w107:dbl, "Screen Aspect Ratio (width in pixels/height in pixels)"=w106:dbl, "Illumination Centre (range: 0 to 1)"=w105:cluster{"x":dbl, "y":dbl})
        n61 = Unbundle(w105) -> ("x"=w112:dbl, "y"=w111:dbl)
        n62 = Format Into String(format string="<aspect>\n%.;%f, %f\n</aspect>\n", initial string=w109, w107, w106) -> (resulting string=w110:string)  [unwired: 1 in, 1 out]
        n63 = Format Into String(format string="<centre>\n%.;%f, %f\n</centre>\n", initial string=w110, w112, w111) -> (resulting string=w104:string)  [unwired: 1 in, 1 out]
      }
    }
    n64 = case shown="False" "Save settings to defaults file" {
      tunnel: w38 -> [w79 w82]
      tunnel: [w79 w81] -> w41
      frame False {
      }
      frame True {
        n65 = Concatenate Strings(w82, "<save/>\n" ("string")) -> (w81:string)
      }
    }
    n66 = Concatenate Strings("<data>\n" ("Data String"), w41, "</data>" ("Data String")) -> (w20:string)
    "message" <- w20
    n67 = String Length(string=w20) -> (length=→"length":i32)
    n68 = String To IP(1:"Remote Host") -> (0:w50:u32)
    n69 = UDP Write(address=w50, port or service name="Remote Port", connection ID=w58, data in=w20, 8:w56) -> (error out=w62:errorcluster, 3:w61:refnum<k16>)  [unwired: 1 out]
  }
  "error out" <- w2
  n70 = case shown="True" w3 {
    frame False {
    }
    frame True {
      n71 = property on="Phase Map" class="IntGraph (strict)"("ZScale.MarkerVals[]"=cluster{dbl, u32}[] [{-3.141, 0}, {0.0, 255}, {3.141, 16777215}] ("Z Scale.Marker Values[]")) -> ()  [unwired: 2 in, 2 out]
    }
  }
  n72 = disable-structure shown="Disabled" {
    disable-tunnel: "Show panel" -> [w163 _]
    frame Disabled {
      n73 = case shown="True" w163 {
        frame False {
          n74 = property class="VI"("Front Panel.Open"=FALSE ("Front Panel Window:Open")) -> ()  [unwired: 2 in, 2 out]
        }
        frame True {
          n75 = property class="VI"("Front Panel.Open"=TRUE ("Front Panel Window:Open")) -> ()  [unwired: 2 in, 2 out]
        }
      }
    }
    frame Enabled {
    }
  }
